vi "AuMT8852B EDR Differential Phase Encoding Extended Results PHASE XRSULT.vi"(5 "Stage":T2(ring), 8 "error in (no error)":errorcluster, 11 "VISA session":refnum<visa-resource-name>) -> (0 "error out":errorcluster, 2 "error code":i32, 3 "VISA session out":refnum<visa-resource-name>, 4 "Results":T1)   [LabVIEW 2017]
doc: "Anritsu MT8852B Bluetooth Tester\n\nReturns the results of the EDR Differential Phase test.\n\nINPUTS\nStage - results of the individual hopping stages of the test.\n\nOUTPUTS\nResults - measurements made during the test."
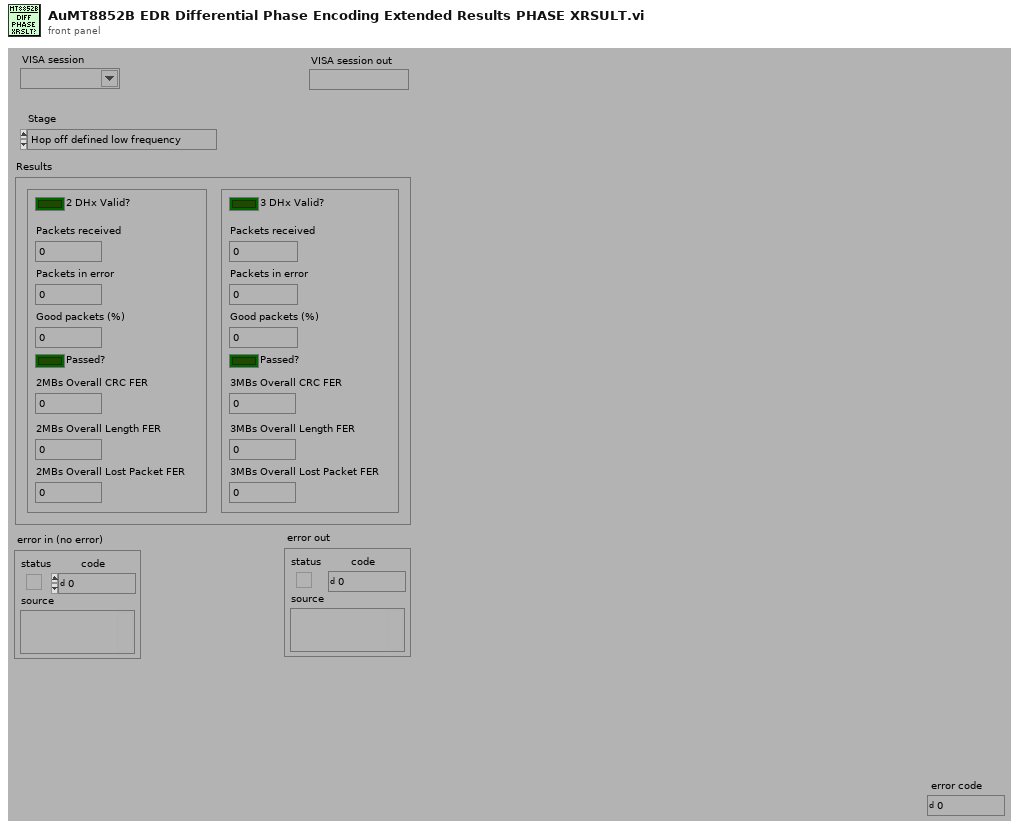
[diagram p1: front panel]
types:
  T1 = cluster{"2 DHx Valid?":bool, "Packets received":u32, "Packets in error":u32, "Passed?":bool, "Good packets (%)":u32, "3 DHx Valid?":bool, "Packets received":u32, "Packets in error":u32, "Passed?":bool, "Good packets (%)":u32, "2MBs Overall CRC FER":u32, "2MBs Overall Length FER":u32, "2MBs Overall Lost Packet FER":u32, "3MBs Overall CRC FER":u32, "3MBs Overall Length FER":u32, "3MBs Overall Lost Packet FER":u32}
  T2 = enum16{"Hop off defined low frequency", "Hop off defined medium frequency", "Hop off defined high frequency", "Hop on any channels"}
  T3 = enum16{"Simulate", "Range check", "Cache", "Query instrument status"}
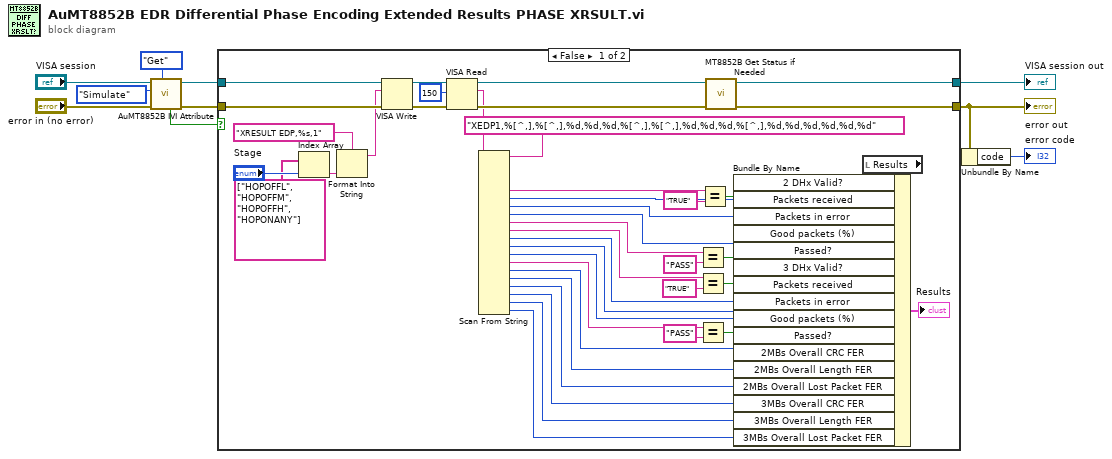
[diagram p0: block diagram]
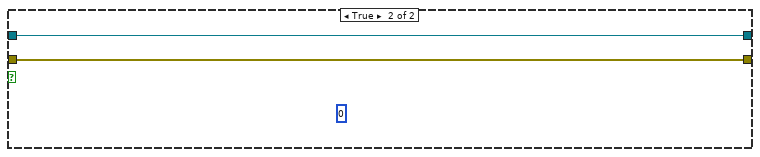
[diagram p2: hidden frame]
diagram:
  n1 = call <instrlib>:"AuMT8852B IVI Attribute.vi"("Set/Get (Set)"=enum16{"Set", "Get"}."Get", "error in (no error)"="error in (no error)", "Flag (Simulate)"=T3."Simulate", "VISA session"="VISA session") -> ("error out"=w7:errorcluster, "VISA session out"=w9:refnum<visa-resource-name>, "Value out"=w3:bool)  [unwired: 5 in]
  n2 = case shown="False" w3 {
    tunnel: [w46 w54] -> w10
    tunnel: [w45 w53] -> w1
    tunnel: w9 -> [w52 w54]
    tunnel: w7 -> [w51 w53]
    frame False {
      n3 = Index Array(array=string[] ["HOPOFFL", "HOPOFFM", "HOPOFFH", "HOPONANY"], index="Stage") -> (element=w34:string)
      n4 = Format Into String(format string="XRESULT EDP,%s,1" ("write buffer (\"\")"), w34) -> (resulting string=w31:string)  [unwired: 2 in, 1 out]
      n5 = VISA Write(VISA resource name=w52, write buffer=w31, error in (no error)=w51) -> (VISA resource name out=w50:refnum<visa-resource-name>, error out=w49:errorcluster)  [unwired: 1 out]
      n6 = VISA Read(VISA resource name=w50, byte count=u32 150 ("byte count (0)"), error in (no error)=w49) -> (VISA resource name out=w44:refnum<visa-resource-name>, read buffer=w29:string, error out=w43:errorcluster)  [unwired: 1 out]
      n7 = Scan From String(format string="XEDP1,%[^,],%[^,],%d,%d,%d,%[^,],%[^,],%d,%d,%d,%[^,],%d,%d,%d,%d,%d,%d" ("Format String"), input string=w29) -> (output 2=w28:string, output 3=w27:i32, output 4=w26:i32, output 5=w25:i32, output 6=w23:string, output 7=w24:string, output 8=w22:i32, output 9=w21:i32, output 10=w20:i32, output 11=w19:string, output 12=w16:i32, output 13=w15:i32, output 14=w14:i32, output 15=w13:i32, output 16=w12:i32, output 17=w11:i32)  [unwired: 20 in, 3 out]
      n8 = Equal?(x=w23, y="PASS") -> (x = y?=w39:bool)
      n9 = Equal?(x=w24, y="TRUE") -> (x = y?=w38:bool)
      n10 = Equal?(x=w19, y="PASS") -> (x = y?=w37:bool)
      n11 = Equal?(x=w28, y="TRUE") -> (x = y?=w42:bool)
      n12 = call <instrlib>:"MT8852B Get Status if Needed.vi"("error in (no error)"=w43, "VISA session"=w44) -> ("error out"=w45:errorcluster, "VISA session out"=w46:refnum<visa-resource-name>)  [unwired: 8 in]
      n13 = local read "Results"() -> (w17:T1)
      n14 = Bundle By Name(cluster=w17, "2 DHx Valid?"=w42, "Packets received"=w27, "Packets in error"=w26, "Good packets (%)"=w25, "Passed?"=w39, "3 DHx Valid?"=w38, "Packets received"=w22, "Packets in error"=w21, "Good packets (%)"=w20, "Passed?"=w37, "2MBs Overall CRC FER"=w16, "2MBs Overall Length FER"=w15, "2MBs Overall Lost Packet FER"=w14, "3MBs Overall CRC FER"=w13, "3MBs Overall Length FER"=w12, "3MBs Overall Lost Packet FER"=w11) -> (→"Results":T1)
    }
    frame True {
      (unwired) u8 0
    }
  }
  "error out" <- w1
  "VISA session out" <- w10
  n15 = Unbundle By Name(w1) -> ("code"=→"error code":i32)
